vi "Eigenvalues.vi"(1 "Number of Rotations (100)":i32, 2 "n":i32, 3 "A":fxp<+/-,32,16>[](array[numeric])) -> (0 "eigenvalues":fxp<+/-,32,16>[](array[numeric]))   [LabVIEW 2020]
panel:
  in  "FXP_type":fxp<+/-,32,16>
  in  "eigenvalue_type":fxp<+/-,32,16>
  in  "near_zero_constant":sgl=1e-36 format="%#_13g"
  in  "A_max":fxp<+/-,32,16>
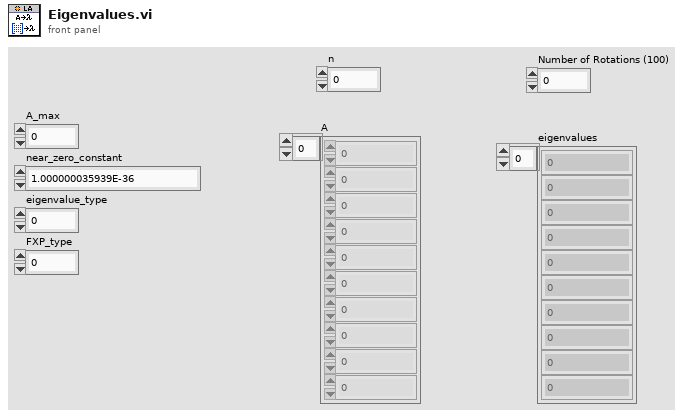
[diagram p1: front panel]
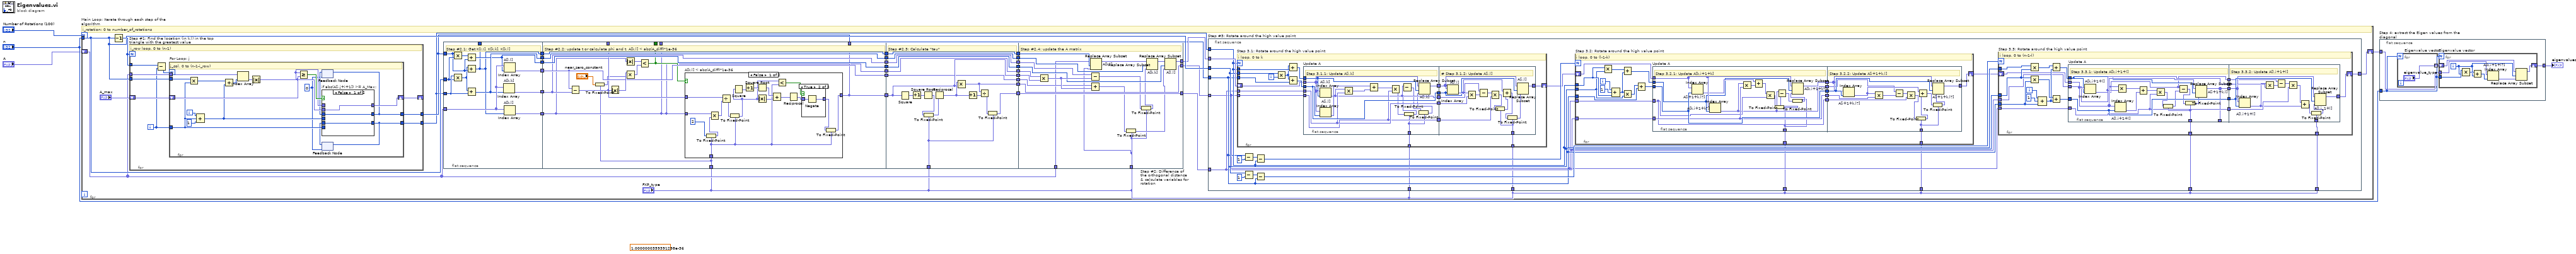
[diagram p0: block diagram]
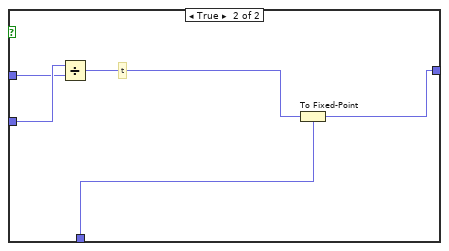
[diagram p3: hidden frame]
diagram:
  (unwired) sgl 1e-36 ("y")
  n1 = for "Main Loop: Iterate through each step of the algorithm" {
    N: "Number of Rotations (100)" -> [_]
    tunnel: "n" -> [w36]
    shift-right: [w7] -> w2
    shift-left: "A" -> [w26]
    # "i_rotation: 0 to number_of_rotations"
    n2 = Decrement(x=w36) -> (x-1=w37:i32)
    n3 = for "Step #1: Find the location (in k,l) in the top triangle with the greatest value" {
      N: w37 -> [_]
      tunnel: w37 -> [w297]
      shift-right: [w301] -> _
      shift-left: "A_max" -> [w299]
      tunnel: [w300] -> w9
      tunnel: [w298] -> w8
      tunnel: w26 -> [w296]
      tunnel: w36 -> [w295]
      i -> [w294]
      # "i_row loop, 0 to (n-1)"
      n4 = Subtract(x=w297, y=w294) -> (x-y=w302:i32)
      n5 = for "For Loop: j" {
        N: w302 -> [_]
        shift-right: [w311] -> w301
        shift-left: w299 -> [w310]
        tunnel: [w303] -> w300
        tunnel: [w307] -> w298
        tunnel: w296 -> [w320]
        tunnel: w294 -> [w309]
        tunnel: w295 -> [w318]
        i -> [w314]
        w304 = 0
        # "j_col, 0 to (n-1-i_row)"
        n6 = Multiply(x=w318, y=w309) -> (x*y=w316:i32)
        n7 = Compound Arithmetic op=ADD(w314, w309, 1 ("value")) -> (w306:i32)
        n8 = Add(x=w316, y=w306) -> (x+y=w315:i32)
        n9 = Index Array(array=w320, index=w315) -> (element=w317:fxp<+/-,32,16>)
        n10 = Absolute Value(x=w317) -> (abs(x)=w312:fxp<+,32,16>)
        n11 = Greater Or Equal?(x=w312, y=w310) -> (x >= y?=w313:bool)
        n12 = feedback #1(w304) -> (w305:i32)
        n13 = feedback #2(w304) -> (w308:i32)
        n14 = case "if abs(A[i,j+i+1]) >= A_Max:" shown="False" w313 {
          tunnel: [w323 w326] -> w311
          tunnel: w312 -> [_ w326]
          tunnel: w310 -> [w323 _]
          tunnel: w309 -> [_ w325]
          tunnel: [w322 w325] -> w307
          tunnel: w308 -> [w322 _]
          tunnel: w306 -> [_ w324]
          tunnel: [w321 w324] -> w303
          tunnel: w305 -> [w321 _]
          frame False {
          }
          frame True {
          }
        }
        n15 = feedback-in #1(w303) -> ()
        n16 = feedback-in #2(w307) -> ()
      }
    }
    n17 = flat-sequence "Step #2: Difference of the orthogonal distance & calculate variables for rotation" {
      tunnel: [w46] -> w33
      tunnel: [w45] -> w32
      tunnel: [w44] -> w31
      tunnel: w8 -> [w50]
      tunnel: w36 -> [w49]
      tunnel: w9 -> [w48]
      tunnel: w26 -> [w47]
      tunnel: [w39] -> w22
      tunnel: [w41] -> w21
      tunnel: [w40] -> w18
      tunnel: [w39] -> _
      tunnel: [w57] -> w30
      tunnel: w33 -> [w59]
      tunnel: w32 -> [w58]
      tunnel: w31 -> [w54]
      tunnel: [w62] -> w23
      tunnel: w22 -> [w62]
      tunnel: w21 -> [w61]
      tunnel: [w61] -> w20
      tunnel: w18 -> [w60]
      tunnel: [w60] -> w17
      tunnel: [w54] -> w15
      tunnel: [w59] -> w13
      tunnel: [w58] -> w11
      tunnel: [w57] -> _
      tunnel: [w56] -> _
      tunnel: [w55] -> _
      tunnel: [w54] -> _
      tunnel: "FXP_type" -> [w51]
      tunnel: w30 -> [w103]
      tunnel: [w103] -> w29
      tunnel: [w102] -> w28
      tunnel: [w93] -> w27
      tunnel: [w101] -> w24
      tunnel: w23 -> [w101]
      tunnel: w20 -> [w100]
      tunnel: [w100] -> w19
      tunnel: w17 -> [w99]
      tunnel: [w99] -> w16
      tunnel: w15 -> [w98]
      tunnel: [w98] -> w14
      tunnel: w13 -> [w97]
      tunnel: [w97] -> w12
      tunnel: w11 -> [w96]
      tunnel: [w96] -> w10
      tunnel: "FXP_type" -> [w91]
      tunnel: [w125] -> w34
      tunnel: [w126] -> w35
      tunnel: w29 -> [w124]
      tunnel: w28 -> [w126]
      tunnel: w27 -> [w125]
      tunnel: w26 -> [w115]
      tunnel: [w116] -> w25
      tunnel: w24 -> [w122]
      tunnel: w19 -> [w121]
      tunnel: w16 -> [w120]
      tunnel: w14 -> [w119]
      tunnel: w12 -> [w118]
      tunnel: w10 -> [w117]
      tunnel: "FXP_type" -> [w108]
      frame #0 {
        # "Step #2.1: Get K[I,I], K[k,k], K[k,l]"
        n18 = Multiply(x=w48, y=w49) -> (x*y=w43:i32)
        n19 = Multiply(x=w50, y=w49) -> (x*y=w42:i32)
        n20 = Add(x=w43, y=w48) -> (x+y=w40:i32)
        n21 = Add(x=w42, y=w48) -> (x+y=w39:i32)
        n22 = Add(x=w42, y=w50) -> (x+y=w41:i32)
        n23 = Index Array "A[k,k]"(array=w47, index=w41) -> (element=w45:fxp<+/-,32,16>)
        n24 = Index Array "A[l,l]"(array=w47, index=w40) -> (element=w46:fxp<+/-,32,16>)
        n25 = Index Array "A[k,l]"(array=w47, index=w39) -> (element=w44:fxp<+/-,32,16>)
      }
      frame #1 {
        # "Step #2.2: update t or calculate phi and t, A[k,l] < abs(A_diff)*1e-36"
        n26 = Subtract(x=w59, y=w58) -> (x-y=w56:fxp<+/-,33,17>)
        n27 = To Fixed-Point(fixed-point type=w51, number="near_zero_constant") -> (fixed-point=w52:fxp<+/-,32,16>)
        n28 = Absolute Value(x=w56) -> (abs(x)=w63:fxp<+,32,16>)
        n29 = Absolute Value(x=w54) -> (abs(x)=w65:fxp<+,32,16>)
        n30 = Multiply(x=w63, y=w52) -> (x*y=w64:fxp<+/-,64,32>)
        n31 = Less?(x=w65, y=w64) -> (x < y?=w55:bool)
        n32 = case "A[k,l] < abs(A_diff)*1e-36" shown="False" w55 {
          tunnel: w54 -> [w82 w90]
          tunnel: w56 -> [w80 w89]
          tunnel: [w67 w87] -> w57
          tunnel: w51 -> [w66 w86]
          frame False {
            n33 = To Fixed-Point(fixed-point type=w66, number=i8 2 ("y")) -> (fixed-point=w71:fxp<+/-,32,16>)
            n34 = Multiply(x=w82, y=w71) -> (x*y=w81:fxp<+/-,64,32>)
            n35 = Divide(x=w80, y=w81) -> (x/y=w70:fxp<+/-,64,49>)
            n36 = To Fixed-Point(fixed-point type=w66, number=w70) -> (fixed-point=w69:fxp<+/-,32,16>)
            n37 = Square(x=w69) -> (x^2=w78:fxp<+,63,31>)
            n38 = Increment(x=w78) -> (x+1=w77:fxp<+,63,31>)
            n39 = Square Root(x=w77) -> (sqrt(x)=w76:fxp<+,64,16>)
            n40 = Absolute Value(x=w69) -> (abs(x)=w79:fxp<+,32,16>)
            n41 = Add(x=w76, y=w79) -> (x+y=w75:fxp<+,64,17>)
            n42 = Less?(x=w69, y=w66) -> (x < y?=w74:bool)
            n43 = Reciprocal(x=w75) -> (1/x=w73:fxp<+,64,48>)
            n44 = case shown="True" w74 {
              tunnel: w73 -> [w83 w85]
              tunnel: [w83 w84] -> w68
              frame False {
              }
              frame True {
                n45 = Negate(x=w85) -> (-x=w84:fxp<+/-,64,49>)
              }
            }
            n46 = To Fixed-Point(fixed-point type=w66, number=w68) -> (fixed-point=w67:fxp<+/-,32,16>)
          }
          frame True {
            # "t"
            n47 = Divide(x=w90, y=w89) -> (x/y=w88:fxp<+/-,64,33>)
            n48 = To Fixed-Point(fixed-point type=w86, number=w88) -> (fixed-point=w87:fxp<+/-,32,16>)
          }
        }
      }
      frame #2 {
        # "Step #2.3: Calculate \"tau\""
        n49 = Square(x=w103) -> (x^2=w105:fxp<+,63,31>)
        n50 = Increment(x=w105) -> (x+1=w104:fxp<+,63,31>)
        n51 = Square Root(x=w104) -> (sqrt(x)=w95:fxp<+,64,16>)
        n52 = To Fixed-Point(fixed-point type=w91, number=w95) -> (fixed-point=w94:fxp<+/-,32,16>)
        n53 = Reciprocal(x=w94) -> (1/x=w107:fxp<+/-,34,18>)
        n54 = Multiply(x=w107, y=w103) -> (x*y=w102:fxp<+/-,64,33>)
        n55 = Increment(x=w107) -> (x+1=w106:fxp<+/-,34,18>)
        n56 = Divide(x=w102, y=w106) -> (x/y=w92:fxp<+/-,64,50>)
        n57 = To Fixed-Point(fixed-point type=w91, number=w92) -> (fixed-point=w93:fxp<+/-,32,16>)
      }
      frame #3 {
        # "Step #2.4: update the A matrix"
        n58 = Multiply(x=w119, y=w124) -> (x*y=w123:fxp<+/-,64,32>)
        n59 = Subtract(x=w117, y=w123) -> (x-y=w110:fxp<+/-,64,32>)
        n60 = Add(x=w118, y=w123) -> (x+y=w112:fxp<+/-,64,32>)
        n61 = Replace Array Subset "A[k,l]"(array=w115, new element=w108, index=w122) -> (w114:fxp<+/-,32,16>[])
        n62 = To Fixed-Point(fixed-point type=w108, number=w112) -> (fixed-point=w111:fxp<+/-,32,16>)
        n63 = To Fixed-Point(fixed-point type=w108, number=w110) -> (fixed-point=w109:fxp<+/-,32,16>)
        n64 = Replace Array Subset "A[k,k]"(array=w114, new element=w109, index=w121) -> (w113:fxp<+/-,32,16>[])
        n65 = Replace Array Subset "A[l,l]"(array=w113, new element=w111, index=w120) -> (w116:fxp<+/-,32,16>[])
      }
    }
    n66 = flat-sequence "Step #3: Rotate around the high value point" {
      tunnel: w8 -> [w139]
      tunnel: w25 -> [w147]
      tunnel: w36 -> [w140]
      tunnel: w35 -> [w135]
      tunnel: w34 -> [w136]
      tunnel: w9 -> [w138]
      tunnel: [w137] -> w7
      tunnel: "FXP_type" -> [w132]
      tunnel: "FXP_type" -> [w131]
      tunnel: "FXP_type" -> [w130]
      tunnel: "FXP_type" -> [w129]
      tunnel: "FXP_type" -> [w128]
      tunnel: "FXP_type" -> [w127]
      frame #0 {
        n67 = for "Step 3.1: Rotate around the high value point" {
          N: w139 -> [_]
          tunnel: w140 -> [w263]
          tunnel: w139 -> [w262]
          tunnel: w135 -> [w257]
          tunnel: w136 -> [w261]
          tunnel: w138 -> [w258]
          shift-right: [w250] -> w134
          shift-left: w147 -> [w256]
          tunnel: w132 -> [w248]
          tunnel: w131 -> [w247]
          i -> [w264]
          # "i loop, 0 to k"
          n68 = Multiply(x=w263, y=w264) -> (x*y=w259:i32)
          n69 = Add(x=w259, y=w262) -> (x+y=w255:i32)
          n70 = Add(x=w259, y=w258) -> (x+y=w260:i32)
          n71 = flat-sequence "Update A" {
            tunnel: w261 -> [w273]
            tunnel: w260 -> [w274]
            tunnel: w257 -> [w271]
            tunnel: w256 -> [w276]
            tunnel: w255 -> [w272]
            tunnel: [w275] -> w254
            tunnel: [w274] -> w253
            tunnel: [w273] -> w252
            tunnel: [w271] -> w251
            tunnel: [w270] -> w249
            tunnel: w248 -> [w265]
            tunnel: w254 -> [w293]
            tunnel: w253 -> [w287]
            tunnel: w252 -> [w292]
            tunnel: w251 -> [w289]
            tunnel: [w286] -> w250
            tunnel: w249 -> [w285]
            tunnel: w247 -> [w280]
            frame #0 {
              # "Step 3.1.1: Update A[i,k]"
              n72 = Index Array "A[i,k]"(array=w276, index=w272) -> (element=w270:fxp<+/-,32,16>)
              n73 = Index Array "A[i,l]"(array=w276, index=w274) -> (element=w278:fxp<+/-,32,16>)
              n74 = Multiply(x=w270, y=w273) -> (x*y=w279:fxp<+/-,64,32>)
              n75 = Add(x=w278, y=w279) -> (x+y=w277:fxp<+/-,64,32>)
              n76 = Multiply(x=w277, y=w271) -> (x*y=w269:fxp<+/-,64,64>)
              n77 = To Fixed-Point(fixed-point type=w265, number=w269) -> (fixed-point=w268:fxp<+/-,32,16>)
              n78 = Subtract(x=w270, y=w268) -> (x-y=w267:fxp<+/-,33,17>)
              n79 = To Fixed-Point(fixed-point type=w265, number=w267) -> (fixed-point=w266:fxp<+/-,32,16>)
              n80 = Replace Array Subset "A[i,k]"(array=w276, new element=w266, index=w272) -> (w275:fxp<+/-,32,16>[])
            }
            frame #1 {
              # "# Step 3.1.2: Update A[i,l]"
              n81 = Index Array "A[i,l]"(array=w293, index=w287) -> (element=w288:fxp<+/-,32,16>)
              n82 = Multiply(x=w288, y=w292) -> (x*y=w291:fxp<+/-,64,32>)
              n83 = Subtract(x=w285, y=w291) -> (x-y=w290:fxp<+/-,64,32>)
              n84 = Multiply(x=w290, y=w289) -> (x*y=w282:fxp<+/-,64,64>)
              n85 = To Fixed-Point(fixed-point type=w280, number=w282) -> (fixed-point=w281:fxp<+/-,32,16>)
              n86 = Add(x=w288, y=w281) -> (x+y=w284:fxp<+/-,33,17>)
              n87 = To Fixed-Point(fixed-point type=w280, number=w284) -> (fixed-point=w283:fxp<+/-,32,16>)
              n88 = Replace Array Subset "A[i,l]"(array=w293, new element=w283, index=w287) -> (w286:fxp<+/-,32,16>[])
            }
          }
        }
        n89 = Subtract(x=w138, y=1) -> (x-y=w146:i32)
        n90 = Subtract(x=w140, y=1) -> (x-y=w142:i32)
        n91 = Subtract(x=w146, y=w139) -> (x-y=w144:i32)
        n92 = Subtract(x=w142, y=w138) -> (x-y=w141:i32)
        n93 = for "Step 3.2: Rotate around the high value point" {
          N: w144 -> [_]
          shift-right: [w217] -> w133
          shift-left: w134 -> [w215]
          tunnel: w139 -> [w213]
          tunnel: w140 -> [w209]
          tunnel: w138 -> [w207]
          tunnel: w136 -> [w205]
          tunnel: w135 -> [w203]
          tunnel: w130 -> [w198]
          tunnel: w129 -> [w197]
          i -> [w212]
          # "i loop, 0 to (l-1-k)"
          n94 = Multiply(x=w213, y=w209) -> (x*y=w211:i32)
          n95 = Compound Arithmetic op=ADD(w212, 1 ("value"), w213) -> (w210:i32)
          n96 = Add(x=w211, y=w210) -> (x+y=w206:i32)
          n97 = Multiply(x=w210, y=w209) -> (x*y=w208:i32)
          n98 = Add(x=w208, y=w207) -> (x+y=w204:i32)
          n99 = flat-sequence "Update A" {
            tunnel: [w232] -> w216
            tunnel: w215 -> [w231]
            tunnel: w206 -> [w225]
            tunnel: w205 -> [w226]
            tunnel: w204 -> [w227]
            tunnel: w203 -> [w224]
            tunnel: [w227] -> w202
            tunnel: [w226] -> w201
            tunnel: [w224] -> w200
            tunnel: [w223] -> w199
            tunnel: w198 -> [w218]
            tunnel: [w246] -> w217
            tunnel: w216 -> [w243]
            tunnel: w202 -> [w245]
            tunnel: w201 -> [w244]
            tunnel: w200 -> [w240]
            tunnel: w199 -> [w238]
            tunnel: w197 -> [w233]
            frame #0 {
              # "Step 3.2.1: Update A[k,i+1+k]"
              n100 = Index Array "A[i+1+k,l?]"(array=w231, index=w227) -> (element=w230:fxp<+/-,32,16>)
              n101 = Index Array "A[k,i+1+k?]"(array=w231, index=w225) -> (element=w223:fxp<+/-,32,16>)
              n102 = Multiply(x=w223, y=w226) -> (x*y=w229:fxp<+/-,64,32>)
              n103 = Add(x=w230, y=w229) -> (x+y=w228:fxp<+/-,64,32>)
              n104 = Multiply(x=w228, y=w224) -> (x*y=w222:fxp<+/-,64,64>)
              n105 = To Fixed-Point(fixed-point type=w218, number=w222) -> (fixed-point=w221:fxp<+/-,32,16>)
              n106 = Subtract(x=w223, y=w221) -> (x-y=w220:fxp<+/-,33,17>)
              n107 = To Fixed-Point(fixed-point type=w218, number=w220) -> (fixed-point=w219:fxp<+/-,32,16>)
              n108 = Replace Array Subset "A[k,i+1+k?]"(array=w231, new element=w219, index=w225) -> (w232:fxp<+/-,32,16>[])
            }
            frame #1 {
              # "Step 3.2.2: Update A[i+1+k,l]"
              n109 = Index Array "A[i+1+k,l?]"(array=w243, index=w245) -> (element=w239:fxp<+/-,32,16>)
              n110 = Multiply(x=w239, y=w244) -> (x*y=w242:fxp<+/-,64,32>)
              n111 = Subtract(x=w238, y=w242) -> (x-y=w241:fxp<+/-,64,32>)
              n112 = Multiply(x=w241, y=w240) -> (x*y=w237:fxp<+/-,64,64>)
              n113 = To Fixed-Point(fixed-point type=w233, number=w237) -> (fixed-point=w236:fxp<+/-,32,16>)
              n114 = Add(x=w239, y=w236) -> (x+y=w235:fxp<+/-,33,17>)
              n115 = To Fixed-Point(fixed-point type=w233, number=w235) -> (fixed-point=w234:fxp<+/-,32,16>)
              n116 = Replace Array Subset "A[i+1+k,l?]"(array=w243, new element=w234, index=w245) -> (w246:fxp<+/-,32,16>[])
            }
          }
        }
        n117 = for "Step 3.3: Rotate around the high value point" {
          N: w141 -> [_]
          tunnel: w140 -> [w164]
          tunnel: w139 -> [w168]
          tunnel: w138 -> [w163]
          shift-right: [w151] -> w137
          shift-left: w133 -> [w159]
          tunnel: w136 -> [w157]
          tunnel: w135 -> [w155]
          tunnel: w128 -> [w149]
          tunnel: w127 -> [w148]
          i -> [w167]
          # "i loop, 0 to (n-1-l)"
          n118 = Multiply(x=w168, y=w164) -> (x*y=w165:i32)
          n119 = Multiply(x=w164, y=w163) -> (x*y=w162:i32)
          n120 = Compound Arithmetic op=ADD(w167, 1 ("value"), w163) -> (w161:i32)
          n121 = Add(x=w165, y=w161) -> (x+y=w158:i32)
          n122 = Add(x=w162, y=w161) -> (x+y=w156:i32)
          n123 = flat-sequence "Update A" {
            tunnel: [w175] -> w160
            tunnel: w159 -> [w180]
            tunnel: w158 -> [w177]
            tunnel: w157 -> [w178]
            tunnel: w156 -> [w179]
            tunnel: w155 -> [w176]
            tunnel: [w179] -> w154
            tunnel: [w178] -> w153
            tunnel: [w176] -> w152
            tunnel: [w175] -> _
            tunnel: [w174] -> w150
            tunnel: w149 -> [w171]
            tunnel: [w196] -> w151
            tunnel: w160 -> [w193]
            tunnel: w154 -> [w195]
            tunnel: w153 -> [w194]
            tunnel: w152 -> [w190]
            tunnel: w150 -> [w187]
            tunnel: w148 -> [w184]
            frame #0 {
              # "Step 3.3.1: Update A[k,i+1+l]"
              n124 = Index Array "A[k,i+1+l]"(array=w180, index=w177) -> (element=w174:fxp<+/-,32,16>)
              n125 = Index Array "A[l,i+1+l]"(array=w180, index=w179) -> (element=w182:fxp<+/-,32,16>)
              n126 = Multiply(x=w174, y=w178) -> (x*y=w183:fxp<+/-,64,32>)
              n127 = Add(x=w183, y=w182) -> (x+y=w181:fxp<+/-,64,32>)
              n128 = Multiply(x=w181, y=w176) -> (x*y=w170:fxp<+/-,64,64>)
              n129 = To Fixed-Point(fixed-point type=w171, number=w170) -> (fixed-point=w169:fxp<+/-,32,16>)
              n130 = Subtract(x=w174, y=w169) -> (x-y=w172:fxp<+/-,33,17>)
              n131 = To Fixed-Point(fixed-point type=w171, number=w172) -> (fixed-point=w173:fxp<+/-,32,16>)
              n132 = Replace Array Subset "A[i+1+k,l]"(array=w180, new element=w173, index=w177) -> (w175:fxp<+/-,32,16>[])
            }
            frame #1 {
              # "Step 3.3.2: Update A[l,i+1+l]"
              n133 = Index Array "A[l,i+1+l]"(array=w193, index=w195) -> (element=w188:fxp<+/-,32,16>)
              n134 = Multiply(x=w188, y=w194) -> (x*y=w192:fxp<+/-,64,32>)
              n135 = Subtract(x=w187, y=w192) -> (x-y=w191:fxp<+/-,64,32>)
              n136 = Multiply(x=w191, y=w190) -> (x*y=w189:fxp<+/-,64,64>)
              n137 = Add(x=w189, y=w188) -> (x+y=w186:fxp<+/-,64,65>)
              n138 = To Fixed-Point(fixed-point type=w184, number=w186) -> (fixed-point=w185:fxp<+/-,32,16>)
              n139 = Replace Array Subset "A[l,i_1+l]"(array=w193, new element=w185, index=w195) -> (w196:fxp<+/-,32,16>[])
            }
          }
        }
      }
    }
  }
  n140 = flat-sequence "Step 4: extract the Eigen values from the diagonal" {
    tunnel: w2 -> [w329]
    tunnel: "n" -> [w328]
    tunnel: [w327] -> w4
    frame #0 {
      n141 = for "Eigenvalue vector" {
        N: w328 -> [_]
        tunnel: ["eigenvalue_type"] -> w330 mode=indexing
      }
      n142 = for "Eigenvalue vector" {
        N: w328 -> [_]
        shift-right: [w337] -> w327
        shift-left: w330 -> [w338]
        tunnel: w329 -> [w336]
        tunnel: w328 -> [w335]
        i -> [w333]
        n143 = Multiply(x=w335, y=w333) -> (x*y=w334:i32)
        n144 = Add(x=w334, y=w333) -> (x+y=w332:i32)
        n145 = Index Array "A[k,i+1+l?]"(array=w336, index=w332) -> (element=w331:fxp<+/-,32,16>)
        n146 = Replace Array Subset(array=w338, new element=w331, index=w333) -> (w337:fxp<+/-,32,16>[])
      }
    }
  }
  "eigenvalues" <- w4
